vi "practiceImageAnalysis - ModulePOS.vi"() -> ()   [LabVIEW 2016]
uses:
  <vilib>/Utility/file.llb/Write Delimited Spreadsheet (DBL).vi
  <vilib>/regexp/Match Regular Expression.xnode
  <vilib>/vision/NI_Vision_Development_Module.lvlib
panel:
  out "Selected subarray":T1(plugin-control)
  in  "Pattern match settings":T2={"Algorithm"=2, "Number of Matches Requested"=1, "Minimum Match Score"=800.0, "SubPixel Accuracy"=TRUE, "Rotation Angle Ranges"=[], "Show Search Area"=FALSE, "Show Result"=TRUE} {"Rotation Angle Ranges"."End" format="%.1f"; "Rotation Angle Ranges"."Start" format="%.1f"; "Minimum Match Score" min=0 max=1000 format="%.2f"; "Number of Matches Requested" min=1; "Algorithm" items=["All", "Low Discrepancy Sampling", "Grayscale Value Pyramid", "Gradients Pyramid"]}
  out "Template":T1(plugin-control)
  in  "Evaluate Set of Fiducials":enum16{"mark B", "mark C"}(ring)
  out "Coordinate array for image capture":dbl[][](array[numeric])
  in  "Coordinate file for image capture":path=path "E:/BNL/XYZstage+Camera_CollectedImages/01-31-2017/FiducialCoordinates-captured.csv"
  out "Review":bool=TRUE
  out "Search running?":bool
  in  "Stop and delete":bool
  out "Images Array":T1[](array[plugin-control])
  in  "error in":errorcluster
  out "error out":errorcluster={"status"=TRUE, "code"=7, "source"="Open File+.vi:Open File"}
  out "Filenames Array":string[](array[string])
  in  "Naming Convention":string="*.png"
  in  "Images Directory":path=path "E:/BNL/XYZstage+Camera_CollectedImages/01-31-2017/Images"
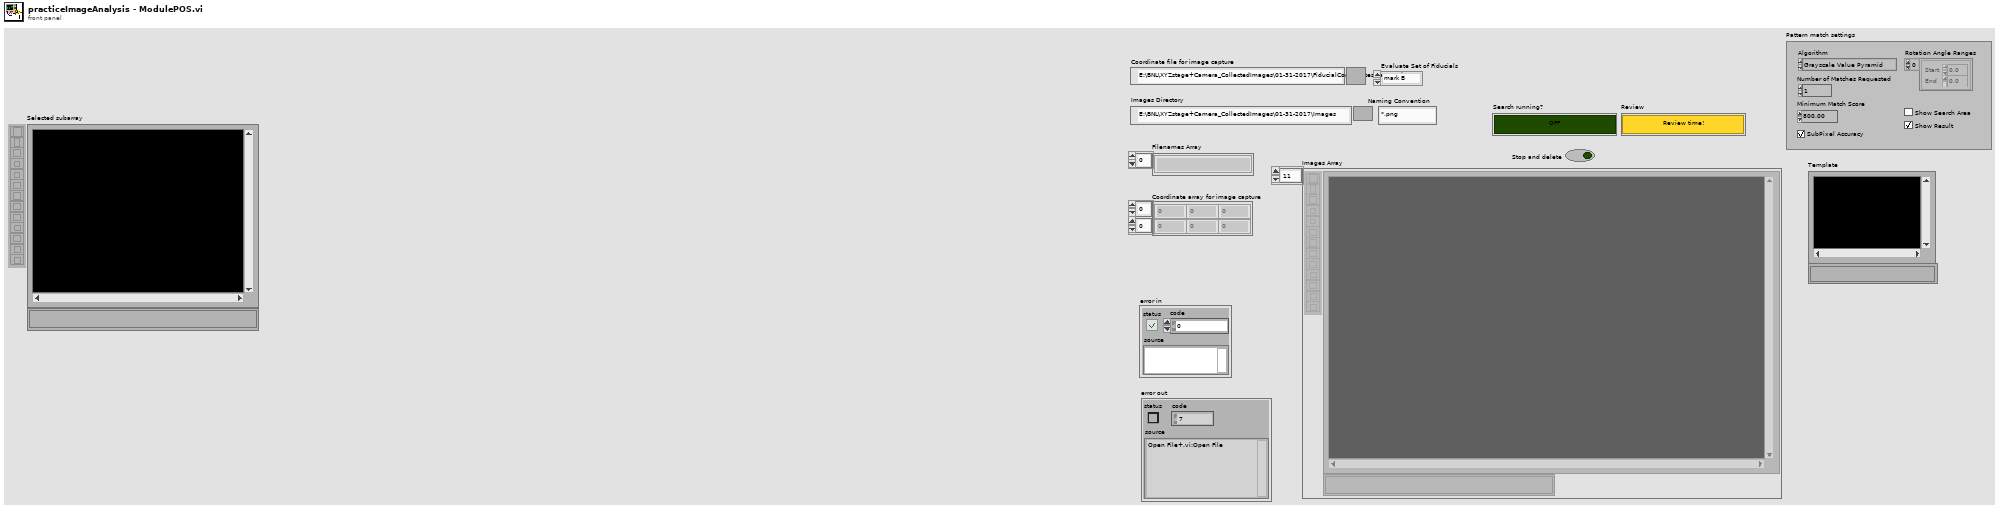
[diagram p1: front panel]
types:
  T1 = typedef "IMAQ Image.ctl" = refnum<image>
  T2 = cluster{"Algorithm":i32, "Number of Matches Requested":i32, "Minimum Match Score":sgl, "SubPixel Accuracy":bool, "Rotation Angle Ranges":cluster{"Start":sgl, "End":sgl}[], "Show Search Area":bool, "Show Result":bool}
  T3 = typedef "Image Type" = u32
  T4 = enum16{"cm", "mm", "pixels [mm/pix]", "pixels [um/pix]"}
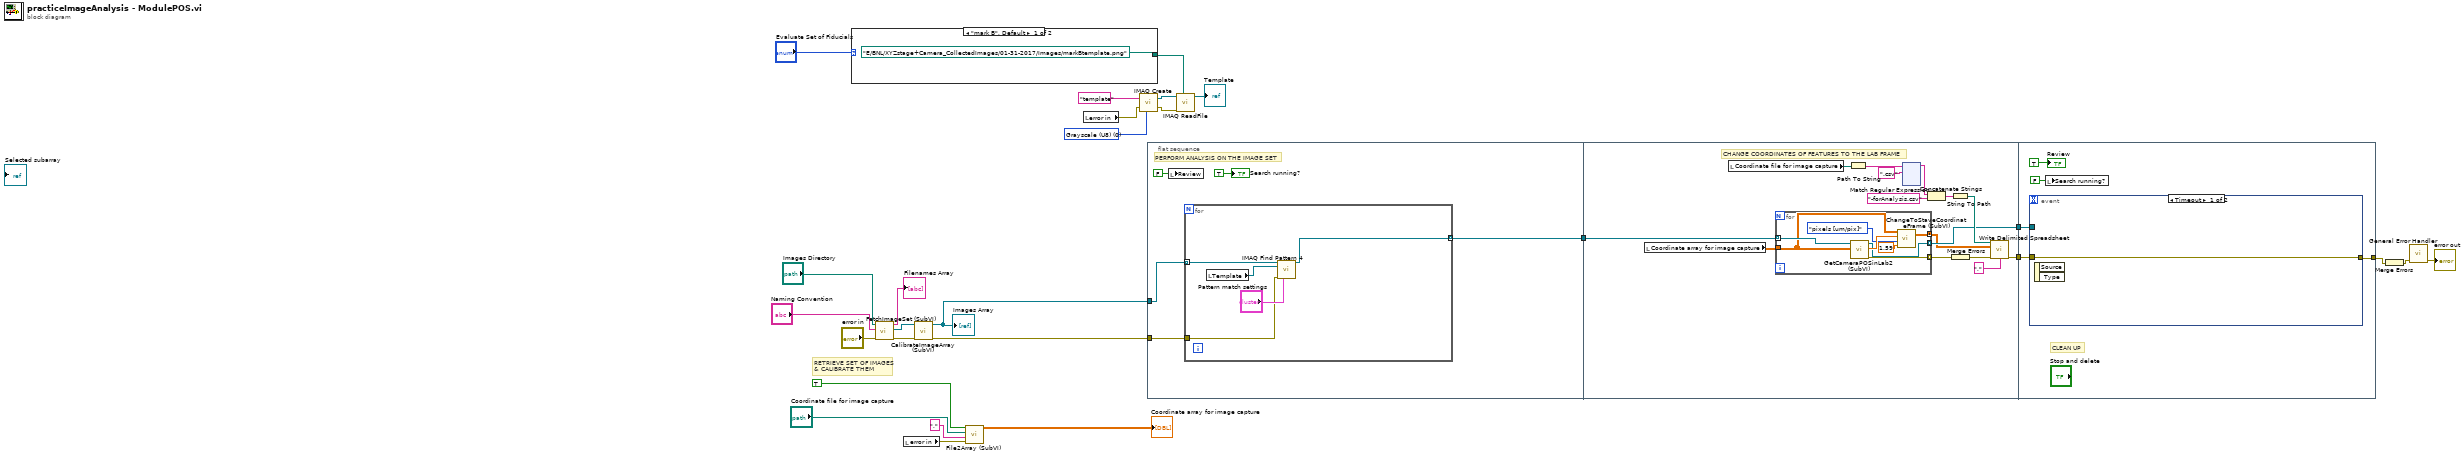
[diagram p0: block diagram]
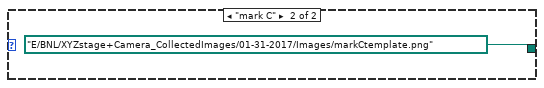
[diagram p2: hidden frame]
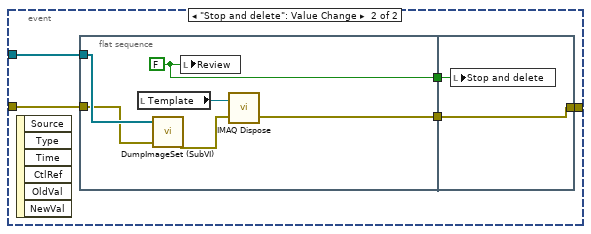
[diagram p3: hidden frame]
diagram:
  w6 = T3 0 items=["Grayscale (U8)", "Grayscale (I16)", "Grayscale (SGL)", "Complex (CSG)", "RGB (U32)", "HSL (U32)", "RGB (U64)", "Grayscale (U16)"] ("Image Type")
  # "RETRIEVE SET OF IMAGES\n& CALIBRATE THEM"
  n1 = case shown="\"mark B\", Default" "Evaluate Set of Fiducials" {
    tunnel: [path "E:/BNL/XYZstage+Camera_CollectedImages/01-31-2017/Images/markBtemplate.png" path "E:/BNL/XYZstage+Camera_CollectedImages/01-31-2017/Images/markCtemplate.png"] -> w5
    frame "mark B", Default {
    }
    frame "mark C" {
    }
  }
  n2 = call "FetchImageSet (SubVI).vi"("error in (no error)"="error in", "Naming Convention"="Naming Convention", "Images Directory"="Images Directory") -> ("error out"=w23:errorcluster, "Image Array"=w24:T1[], "Filenames Array"=→"Filenames Array":string[])  [unwired: 6 in]
  n3 = local read "error in"() -> (w15:errorcluster)
  n4 = call "CalibrateImageArray (SubVI).vi"("error in (no error)"=w23, "Image Array"=w24) -> ("error out"=w20:errorcluster, "Calibrated Image Array"=w19:T1[])  [unwired: 7 in]
  "Images Array" <- w19
  n5 = call "File2Array (SubVI).vi"("error in (no error) in"=w15, "File delimiter"=",", "Source array file"="Coordinate file for image capture", "Load array from file?"=TRUE) -> ("Loaded array"=→"Coordinate array for image capture":dbl[][])  [unwired: 6 in, 1 out]
  n6 = local read "error in"() -> (w8:errorcluster)
  n7 = call "IMAQ Create"("Image Name"="template", "Image Type"=w6, "error in (no error)"=w8) -> ("New Image"=w10:T1, "error out"=w7:errorcluster)  [unwired: 2 in]
  n8 = flat-sequence {
    tunnel: w20 -> [w31]
    tunnel: w19 -> [w32]
    tunnel: [w30] -> w3
    tunnel: [w43] -> w13
    tunnel: w3 -> [w42]
    tunnel: [w41] -> w2
    tunnel: w13 -> [w178]
    tunnel: w2 -> [w179]
    tunnel: [w177] -> w1
    frame #0 {
      # "PERFORM ANALYSIS ON THE IMAGE SET"
      n9 = local write "Review"(FALSE ("Review")) -> ()
      n10 = for {
        tunnel: w32 -> [w39] mode=indexing
        tunnel: w31 -> [w36]
        tunnel: [w35] -> w30 mode=indexing
        n11 = local read "Template"() -> (w38:T1)
        n12 = call "IMAQ Find Pattern 4"("Image"=w39, "Template"=w38, "error in"=w36, "Settings"="Pattern match settings") -> ("Image Out"=w35:T1)  [unwired: 5 in, 6 out]
      }
      "Search running?" <- TRUE ("Search running?")
    }
    frame #1 {
      # "CHANGE COORDINATES OF FEATURES TO THE LAB FRAME"
      n13 = local read "Coordinate array for image capture"() -> (w54:dbl[][])
      n14 = local read "Coordinate file for image capture"() -> (w52:path)
      n15 = for {
        tunnel: w54 -> [w169]
        tunnel: [w173] -> w53 mode=indexing
        tunnel: [w172] -> w40 mode=concatenating
        tunnel: w42 -> [w171] mode=indexing
        tunnel: [w170] -> w41 mode=indexing
        n16 = call "GetCameraPOSinLab2 (SubVI).vi"("Loaded array"=w169, "Refnum in"=w171) -> ("error out"=w173:errorcluster, "Image coordinates in lab frame"=w176:dbl[], "Refnum out"=w170:T1)  [unwired: 7 in]
        n17 = call "ChangeToStaveCoordinateFrame (SubVI).vi"("Loaded array (image frame)"=w169, "Image Origin in XYZ Stage Coords [mm]"=w176, "Units"=T4."pixels [um/pix]", "Pixel resolution"=1.59) -> ("Array (stage frame, mm)"=w172:dbl[][])  [unwired: 2 in]
      }
      n18 = Path To String(path=w52) -> (string=w50:string)
      n19 = xnode "Match Regular Expression"("input string"=w50, "regular expression"=".csv") -> ("before match"=w48:string)  [unwired: 4 in, 4 out]
      n20 = Concatenate Strings(w48, "-forAnalysis.csv" ("name or relative path")) -> (w47:string)
      n21 = String To Path(string=w47) -> (path=w45:path)
      n22 = Merge Errors(w53) -> (w44:errorcluster)
      n23 = call-poly <vilib>:"Write Delimited Spreadsheet.vi"("file path (dialog if empty)"=w45, "2D data"=w40, "error in (no error)"=w44, "delimiter (\\t)"="," ("delimiter (\\t)")) -> ("error out"=w43:errorcluster)  [unwired: 10 in, 1 out]
    }
    frame #2 {
      # "CLEAN UP"
      n24 = event shown="[0] Timeout" {
        selector: _ -> [_ _]
        dyn-events: _ -> [_ _]
        timeout: _ -> [_ _]
        tunnel: w179 -> [_ w186]
        tunnel: w178 -> [w182 w185]
        tunnel: [w182 w183] -> w177
        event Timeout {
          n25 = event-data() -> ()  [unwired: 1 in, 2 out]
        }
        event "Stop and delete": Value Change {
          n26 = event-data() -> ()  [unwired: 1 in, 6 out]
          n27 = flat-sequence {
            tunnel: [w192] -> w187
            tunnel: w186 -> [w190]
            tunnel: w185 -> [w189]
            tunnel: [w188] -> w184
            tunnel: w187 -> [w195]
            tunnel: w184 -> [w194]
            tunnel: [w194] -> w183
            frame #0 {
              w192 = FALSE ("Review")
              n28 = local read "Template"() -> (w193:T1)
              n29 = call "DumpImageSet (SubVI).vi"("error in (no error)"=w189, "Calibrated Image Array"=w190) -> ("error out"=w191:errorcluster)  [unwired: 6 in]
              n30 = local write "Review"(w192) -> ()
              n31 = call "IMAQ Dispose"("Image"=w193, "error in (no error)"=w191) -> ("error out"=w188:errorcluster)  [unwired: 4 in]
            }
            frame #1 {
              n32 = local write "Stop and delete"(w195) -> ()
            }
          }
        }
      }
      n33 = local write "Search running?"(FALSE ("Search running?")) -> ()
      "Review" <- TRUE ("Review")
    }
  }
  n34 = call "IMAQ ReadFile"("File Path"=w5, "error in (no error)"=w7, "Image"=w10) -> ("Image Out"=→"Template":T1)  [unwired: 4 in, 4 out]
  n35 = Merge Errors(w1) -> (w14:errorcluster)
  n36 = call <vilib>:"General Error Handler.vi"("error in (no error)"=w14) -> ("error out"=→"error out":errorcluster)  [unwired: 10 in, 4 out]
